vi "get_params.vi"(8 "error in (no error)":errorcluster caption="entrée d'erreur (pas d'erreur)", 11 "LocallyLinearEmbedding.lvclass 2":refnum<class "LocallyLinearEmbedding.lvclass">) -> (0 "error out":errorcluster caption="sortie d'erreur", 3 "LocallyLinearEmbedding.lvclass":refnum<class "LocallyLinearEmbedding.lvclass">)   [LabVIEW 2020, in "LocallyLinearEmbedding.lvclass"]
uses:
  LocallyLinearEmbedding.lvclass
  LocallyLinearEmbedding.lvclass/LocallyLinearEmbedding.ctl
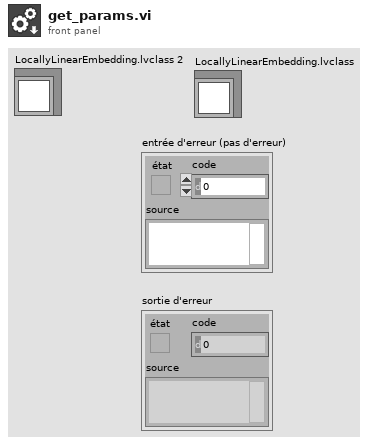
[diagram p1: front panel]
types:
  T1 = typedef "locally_linear_embedding_params.ctl" = cluster{"n_neighbors":dbl, "n_components":dbl, "reg":dbl, "eigen_solver":string, "tol":dbl, "max_iter":dbl, "method":string, "hessian_tol":dbl, "modified_tol":dbl, "neighbors_algorithm":string, "random_state":dbl, "n_jobs":dbl}
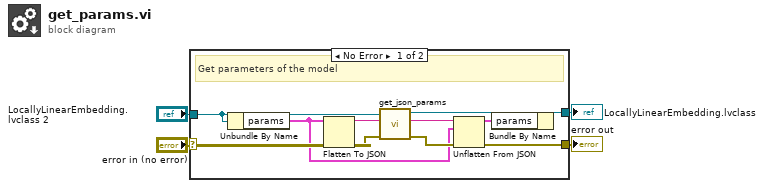
[diagram p0: block diagram]
diagram:
  n1 = case shown="No Error" "error in (no error)" {
    selector: "error in (no error)" -> [w13 w16]
    tunnel: [w5 w16] -> w3
    tunnel: "LocallyLinearEmbedding.lvclass 2" -> [w10 w17]
    tunnel: [w7 w17] -> w1
    frame No Error {
      # "Get parameters of the model"
      n2 = Unbundle By Name(w10) -> ("params"=w9:T1)
      n3 = Flatten To JSON(anything=w9, error in (no error)=w13) -> (JSON string=w12:string, 11:w11:errorcluster)  [unwired: 1 in]
      n4 = call-dynamic "get_json_params.vi"("error in (no error)"=w11, "format"=w12, "Model en entrée"=w10) -> ("error out"=w14:errorcluster, "valeur renvoyée"=w15:string, "Model en sortie"=w8:refnum<class "LocallyLinearEmbedding.lvclass">)  [unwired: 6 in]
      n5 = Unflatten From JSON(JSON string=w15, type and defaults=w9, error in (no error)=w14) -> (value=w6:T1, error out=w5:errorcluster)  [unwired: 4 in]
      n6 = Bundle By Name(cluster=w8, "params"=w6) -> (w7:refnum<class "LocallyLinearEmbedding.lvclass">)
    }
    frame Error {
    }
  }
  "error out" <- w3
  "LocallyLinearEmbedding.lvclass" <- w1
